vi "Servo Example.vi"() -> ()   [LabVIEW 2015, in "LabVIEW Interface for Arduino.lvlib"]
doc: "An example using two servos with the LabVIEW Interface for Arduino."
uses:
  <vilib>/LabVIEW Interface for Arduino/LabVIEW Interface for Arduino.lvlib
panel:
  in  "Speed":u8=1
  in  "Stop":bool
  out "Servo 1":dbl(knob) scale=0.0..180.0
  out "Servo 0":dbl(knob) scale=0.0..180.0
  in  "Servo 1 Angle Input":u8
  in  "Servo 0 Sweep Max Angle":u8=180
  in  "Number of Servos":u8=2
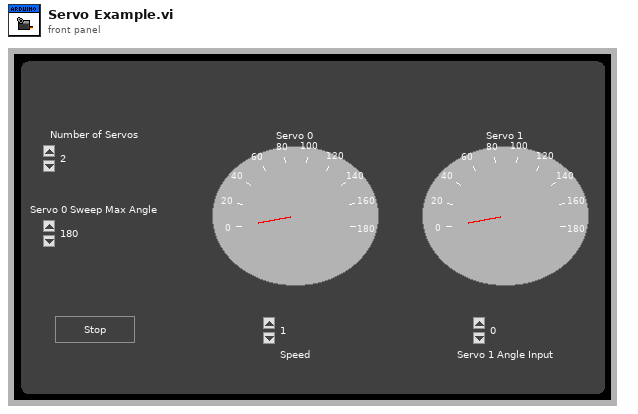
[diagram p1: front panel]
types:
  T1 = typedef "LabVIEW Interface for Arduino.lvlib/Arduino Resource.ctl" = cluster{"VISA resource":refnum<visa-resource-name>, "Board Type":T2, "Connection Type":enum8{"USB / Serial"}, "Bytes Per Packet (15)":u8}
  T2 = typedef "LabVIEW Interface for Arduino.lvlib/Board Type.ctl" = enum16{"Uno", "Dimuelanove w/Atmega 328", "Mega 2560"}
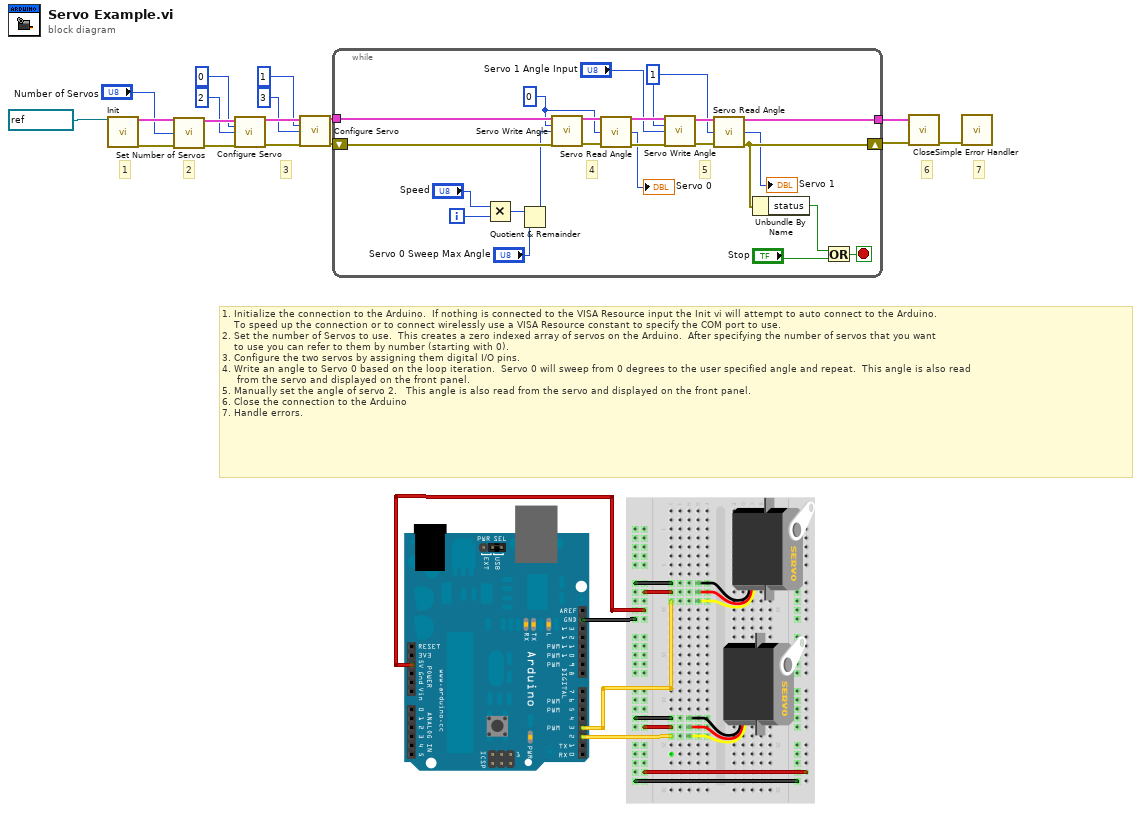
[diagram p0: block diagram]
diagram:
  # "1. Initialize the connection to the Arduino.  If nothing is connected to the VISA Resource input the Init vi will attempt to auto connect to the Arduino.\n    To speed up the connection or to connect wirelessly use a VISA Resource constant to specify the COM port to use.\n2. Set the number of Servos to use.  This creates a zero indexed array of servos on the Arduino.  After specifying the number of servos that you want \n    to use you can refer to them by number (starting with 0).\n3. Configure the two servos by assigning them digital I/O pins.\n4. Write an angle to Servo 0 based on the loop iteration.  Servo 0 will sweep from 0 degrees to the user specified angle and repeat.  This angle is also read\n     from the servo and displayed on the front panel.\n5. Manually set the angle of servo 2.   This angle is also read from the servo and displayed on the front panel.\n6. Close the connection to the Arduino\n7. Handle errors."
  # "7"
  # "6"
  # "3"
  # "2"
  # "1"
  n1 = call <vilib>:"Init.vi"("VISA resource"=refnum<visa-resource-name> "COM4") -> ("Arduino Resource"=w17:T1, "error out"=w16:errorcluster)  [unwired: 17 in]
  n2 = call <vilib>:"Set Number of Servos.vi"("Arduino Resource"=w17, "Number Of Servos (1)"="Number of Servos", "error in"=w16) -> ("Arduino Resource"=w14:T1, "error out"=w13:errorcluster)  [unwired: 11 in]
  n3 = call <vilib>:"Configure Servo.vi"("Arduino Resource"=w14, "Servo Number (0)"=u8 0 ("Servo Number"), "DIO Pin (2)"=u8 2 ("Servo Number"), "error in"=w13) -> ("Arduino Resource"=w12:T1, "error out"=w11:errorcluster)  [unwired: 10 in]
  n4 = call <vilib>:"Configure Servo.vi"("Arduino Resource"=w12, "Servo Number (0)"=u8 1 ("Servo Number"), "DIO Pin (2)"=u8 3 ("Servo Number"), "error in"=w11) -> ("Arduino Resource"=w6:T1, "error out"=w5:errorcluster)  [unwired: 10 in]
  n5 = while {
    tunnel: w6 -> [w40]
    tunnel: [w34] -> w3
    shift-right: [w28] -> w4
    shift-left: w5 -> [w38]
    i -> [w19]
    stop <- w27 stop-if-true
    w25 = u8 1 ("Servo Number")
    w24 = u8 0 ("Servo Number")
    # "5"
    # "4"
    n6 = Multiply(x="Speed", y=w19) -> (x*y=w20:i32)
    n7 = Quotient & Remainder(x=w20, y="Servo 0 Sweep Max Angle") -> (x-y*floor(x/y)=w31:i32)  [unwired: 1 out]
    n8 = call <vilib>:"Servo Write Angle.vi"("Arduino Resource"=w40, "Servo Number"=w24, "Angle (Degrees)"=w31, "error in"=w38) -> ("Arduino Resource"=w39:T1, "error out"=w37:errorcluster)  [unwired: 10 in]
    n9 = call <vilib>:"Servo Read Angle.vi"("Arduino Resource"=w39, "Servo Number"=w24, "error in"=w37) -> ("Arduino Resource"=w32:T1, "Angle (Degrees)"=→"Servo 0":u8, "error out"=w36:errorcluster)  [unwired: 10 in]
    n10 = call <vilib>:"Servo Write Angle.vi"("Arduino Resource"=w32, "Servo Number"=w25, "Angle (Degrees)"="Servo 1 Angle Input", "error in"=w36) -> ("Arduino Resource"=w33:T1, "error out"=w35:errorcluster)  [unwired: 10 in]
    n11 = call <vilib>:"Servo Read Angle.vi"("Arduino Resource"=w33, "Servo Number"=w25, "error in"=w35) -> ("Arduino Resource"=w34:T1, "Angle (Degrees)"=→"Servo 1":u8, "error out"=w28:errorcluster)  [unwired: 10 in]
    n12 = Unbundle By Name(w28) -> ("status"=w26:bool)
    n13 = Or(x=w26, y="Stop") -> (x .or. y?=w27:bool)
  }
  n14 = call <vilib>:"Close.vi"("Arduino Resource"=w3, "error in"=w4) -> ("error out"=w1:errorcluster)  [unwired: 13 in]
  n15 = call <vilib>:"Simple Error Handler.vi"("error in (no error)"=w1) -> ()  [unwired: 4 in, 5 out]
